vi "Motor Controls Ret. Val. Interpreter.vi"(8 "error in":errorcluster, 11 "Command Return":string) -> (0 "error out":errorcluster, 3 "Numeric Output":dbl)   [LabVIEW 2020]
uses:
  <vilib>/regexp/Match Regular Expression.xnode
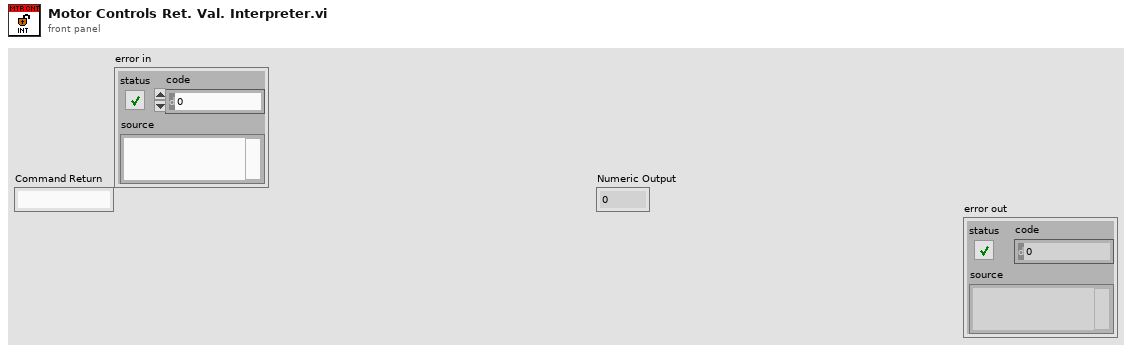
[diagram p1: front panel]
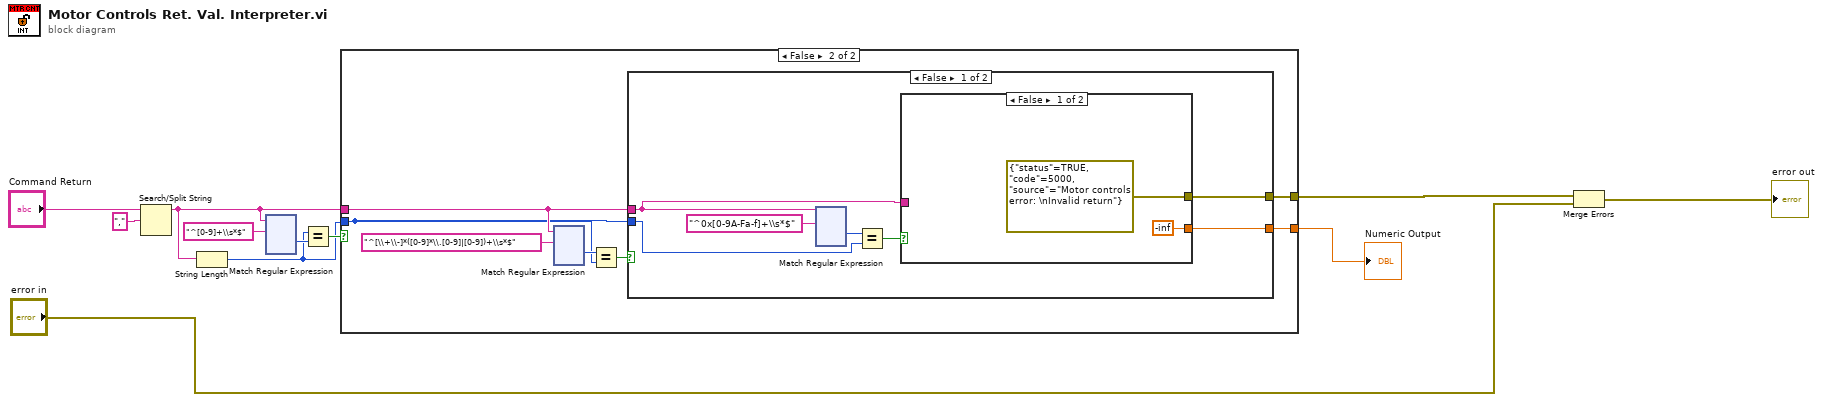
[diagram p0: block diagram]
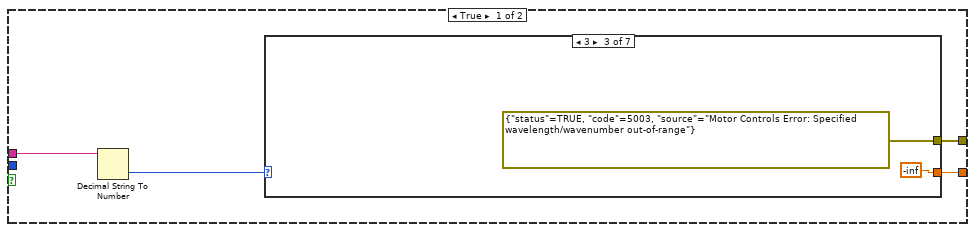
[diagram p2: hidden frame]
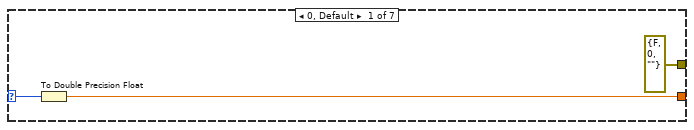
[diagram p3: hidden frame]
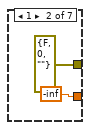
[diagram p4: hidden frame]
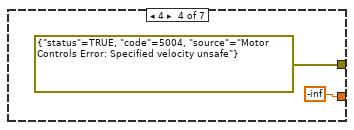
[diagram p5: hidden frame]
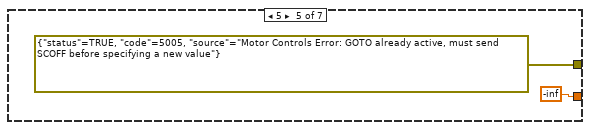
[diagram p6: hidden frame]
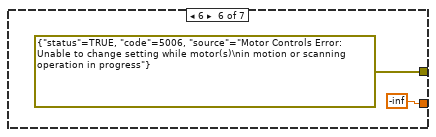
[diagram p7: hidden frame]
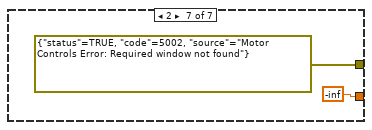
[diagram p8: hidden frame]
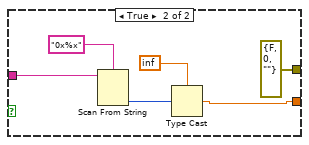
[diagram p9: hidden frame]
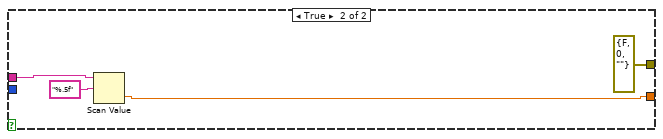
[diagram p10: hidden frame]
diagram:
  n1 = Search/Split String(string="Command Return", search string/char (-)=",") -> (substring before match=w7:string)  [unwired: 1 in, 2 out]
  n2 = String Length(string=w7) -> (length=w6:i32)
  n3 = xnode "Match Regular Expression"("input string"=w7, "regular expression"="^[0-9]+\\s*$") -> ("offset past match"=w9:i32)  [unwired: 4 in, 4 out]
  n4 = Equal?(x=w6, y=w9) -> (x = y?=w8:bool)
  n5 = case shown="False" w8 {
    tunnel: w7 -> [w15 w36]
    tunnel: w6 -> [_ w31]
    tunnel: [w13 w33] -> w3
    tunnel: [w12 w32] -> w4
    frame True {
      n6 = Decimal String To Number(string=w15) -> (number=w14:i32)  [unwired: 2 in, 1 out]
      n7 = case shown="3" w14 {
        selector: w14 -> [w18 _ _ _ _ _ _]
        tunnel: [errorcluster {"status"=FALSE, "code"=0, "source"=""} ("error constant") errorcluster {"status"=FALSE, "code"=0, "source"=""} ("error constant") errorcluster {"status"=TRUE, "code"=5003, "source"="Motor Controls Error: Specified wavelength/wavenumber out-of-range"} ("error constant") errorcluster {"status"=TRUE, "code"=5004, "source"="Motor Controls Error: Specified velocity unsafe"} ("error constant") errorcluster {"status"=TRUE, "code"=5005, "source"="Motor Controls Error: GOTO already active, must send SCOFF before specifying a new value"} ("error constant") errorcluster {"status"=TRUE, "code"=5006, "source"="Motor Controls Error: Unable to change setting while motor(s)\nin motion or scanning operation in progress"} ("error constant") errorcluster {"status"=TRUE, "code"=5002, "source"="Motor Controls Error: Required window not found"} ("error constant")] -> w13
        tunnel: [w17 -inf -inf -inf -inf -inf -inf] -> w12
        frame 0, Default {
          n8 = To Double Precision Float(number=w18) -> (double precision float=w17:dbl)
        }
        frame 1 {
        }
        frame 3 {
        }
        frame 4 {
        }
        frame 5 {
        }
        frame 6 {
        }
        frame 2 {
        }
      }
    }
    frame False {
      n9 = xnode "Match Regular Expression"("input string"=w36, "regular expression"="^[\\+\\-]*([0-9]*\\.[0-9]|[0-9])+\\s*$") -> ("offset past match"=w34:i32)  [unwired: 4 in, 4 out]
      n10 = Equal?(x=w34, y=w31) -> (x = y?=w35:bool)
      n11 = case shown="False" w35 {
        tunnel: w36 -> [w40 w170]
        tunnel: [w39 w168] -> w32
        tunnel: [w38 errorcluster {"status"=FALSE, "code"=0, "source"=""} ("error constant")] -> w33
        tunnel: w31 -> [w41 _]
        frame False {
          n12 = xnode "Match Regular Expression"("input string"=w40, "regular expression"="^0x[0-9A-Fa-f]+\\s*$") -> ("offset past match"=w42:i32)  [unwired: 4 in, 4 out]
          n13 = Equal?(x=w42, y=w41) -> (x = y?=w43:bool)
          n14 = case shown="False" w43 {
            tunnel: w40 -> [_ w52]
            tunnel: [-inf w48] -> w39
            tunnel: [errorcluster {"status"=TRUE, "code"=5000, "source"="Motor controls error: \nInvalid return"} ("error constant") errorcluster {"status"=FALSE, "code"=0, "source"=""} ("error constant")] -> w38
            frame False {
            }
            frame True {
              n15 = Scan From String(format string="0x%x", input string=w52) -> (output 1=w50:u32)  [unwired: 3 in, 3 out]
              n16 = Type Cast(type=inf, x=w50) -> (*(type *) &x=w48:dbl)
            }
          }
        }
        frame True {
          n17 = Scan Value(string=w170, format string="%.5f") -> (value=w168:dbl)  [unwired: 1 in, 1 out]
        }
      }
    }
  }
  "Numeric Output" <- w4
  n18 = Merge Errors(w3, "error in") -> (→"error out":errorcluster)
